vi "SelectFullRow.vi"(8 "error in (no error)":errorcluster, 9 "Coords":T1, 10 "Button":u16, 11 "Table in":refnum<vi>) -> (0 "error out":errorcluster, 3 "Discard?":bool)   [LabVIEW 2017, in "Client.lvlib" / "UI_API.lvlib"]
uses:
  UI_API.lvlib
  <vilib>/Utility/miscctls.llb/LVPoint32TypeDef.ctl
  <vilib>/Utility/miscctls.llb/LVRowAndColumnTypeDef.ctl
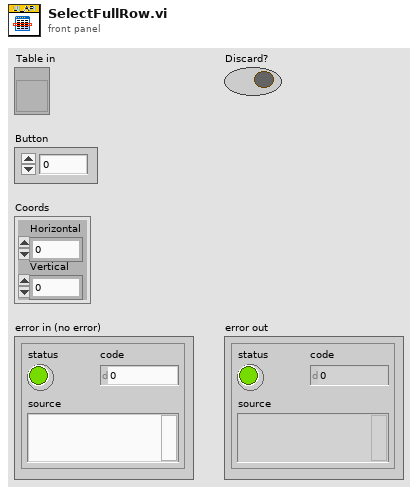
[diagram p1: front panel]
types:
  T1 = typedef "LVPoint32TypeDef.ctl" = cluster{"Horizontal":i32, "Vertical":i32}
  T2 = typedef "LVRowAndColumnTypeDef.ctl" = cluster{"Row":i32, "Column":i32}
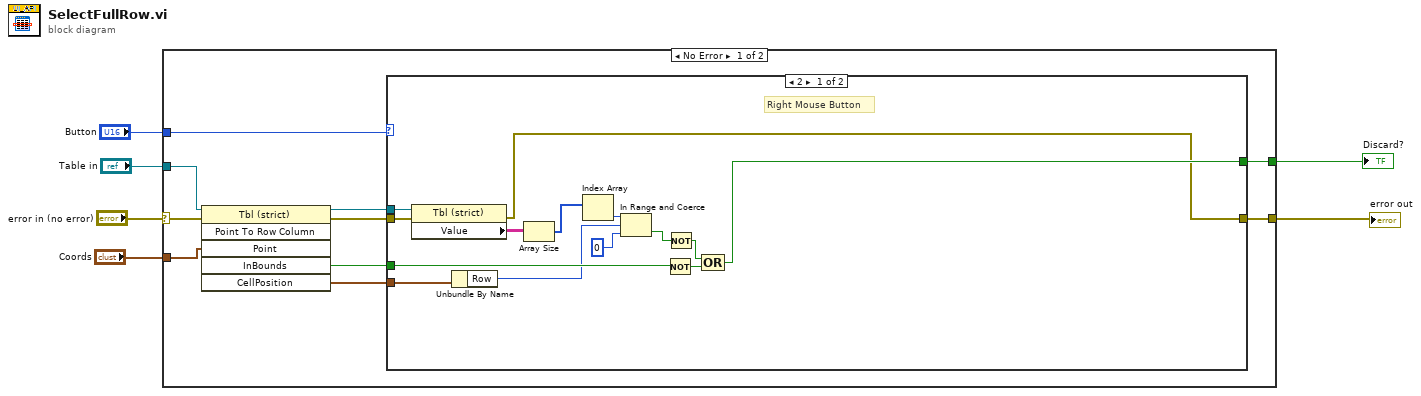
[diagram p0: block diagram]
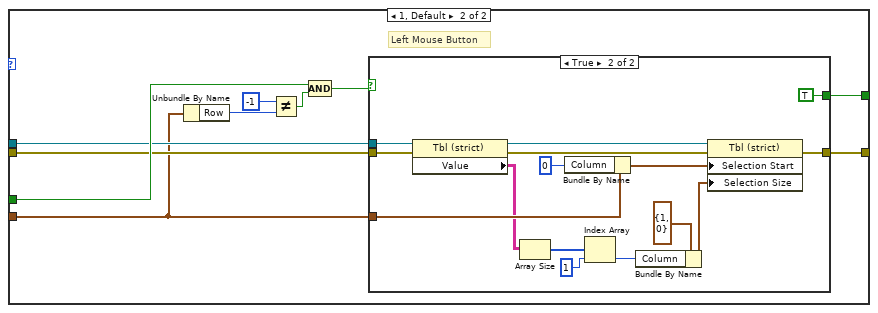
[diagram p2: hidden frame]
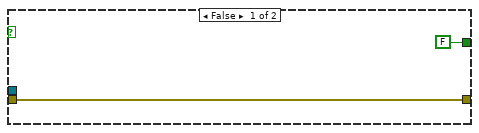
[diagram p3: hidden frame]
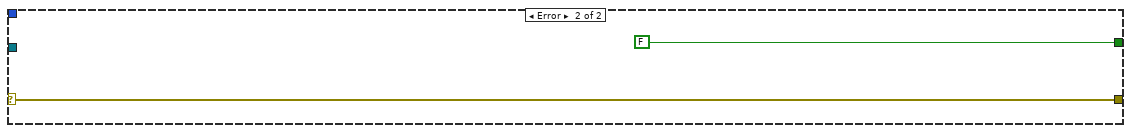
[diagram p4: hidden frame]
diagram:
  n1 = case shown="No Error" "error in (no error)" {
    selector: "error in (no error)" -> [w11 w59]
    tunnel: "Button" -> [w7 _]
    tunnel: "Coords" -> [w13 _]
    tunnel: "Table in" -> [w12 _]
    tunnel: [w10 w59] -> w2
    tunnel: [w9 FALSE ("Discard?")] -> w1
    frame No Error {
      n2 = invoke class="Tbl (strict)" method="Point To Row Column"(reference=w12, error in=w11, "Point"=w13) -> (reference out=w15:refnum<vi>, error out=w14:errorcluster, "InBounds"=w16:bool, "CellPosition"=w8:T2)  [unwired: 3 in, 2 out]
      n3 = case shown="2" w7 {
        tunnel: w16 -> [w30 w40]
        tunnel: w15 -> [w27 w39]
        tunnel: w14 -> [w26 w38]
        tunnel: [w18 w37] -> w10
        tunnel: [w28 w36] -> w9
        tunnel: w8 -> [w23 w34]
        frame 2 {
          # "Right Mouse Button"
          n4 = property class="Tbl (strict)"(reference=w27, error in=w26) -> (error out=w18:errorcluster, "Value"=w25:string[][])  [unwired: 1 out]
          n5 = Unbundle By Name(w23) -> ("Row"=w22:i32)
          n6 = Array Size(array=w25) -> (size(s)=w21:i32[])
          n7 = Index Array(array=w21) -> (element=w17:i32)  [unwired: 1 in]
          n8 = In Range and Coerce(upper limit=w17, x=w22, lower limit=0) -> (In Range?=w20:bool)  [unwired: 1 out]
          n9 = Not(x=w30) -> (.not. x?=w29:bool)
          n10 = Not(x=w20) -> (.not. x?=w19:bool)
          n11 = Compound Arithmetic op=OR(w19, w29) -> (w28:bool)
        }
        frame 1, Default {
          # "Left Mouse Button"
          n12 = Unbundle By Name(w34) -> ("Row"=w33:i32)
          n13 = Not Equal?(x=-1, y=w33) -> (x != y?=w31:bool)
          n14 = Compound Arithmetic op=AND(w40, w31) -> (w35:bool)
          n15 = case shown="True" w35 {
            tunnel: w34 -> [_ w55]
            tunnel: w39 -> [_ w50]
            tunnel: w38 -> [w42 w49]
            tunnel: [w42 w52] -> w37
            tunnel: [FALSE ("Discard?") TRUE ("Discard?")] -> w36
            frame False {
            }
            frame True {
              n16 = property class="Tbl (strict)"(reference=w50, error in=w49) -> (reference out=w47:refnum<vi>, error out=w48:errorcluster, "Value"=w46:string[][])
              n17 = Array Size(array=w46) -> (size(s)=w45:i32[])
              n18 = Bundle By Name(cluster=w55, "Column"=0) -> (w57:T2)
              n19 = Index Array(array=w45, index=1) -> (element=w44:i32)
              n20 = Bundle By Name(cluster=T2 {"Row"=1, "Column"=0} ("Selection Size"), "Column"=w44) -> (w53:T2)
              n21 = property class="Tbl (strict)"(reference=w47, error in=w48, "Selection Start"=w57, "Selection Size"=w53) -> (error out=w52:errorcluster)  [unwired: 1 out]
            }
          }
        }
      }
    }
    frame Error {
    }
  }
  "Discard?" <- w1
  "error out" <- w2
